vi "MT Set Axis Halt All.vi"() -> (3 "function return":i32)   [LabVIEW 2014, in "MT_API.lvlib"]
doc: "MT_API INT32 __stdcall MT_Set_Axis_Halt_All(void);"
uses:
  MT_API.lvlib
  MT_API.dll
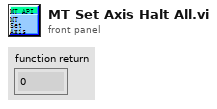
[diagram p1: front panel]
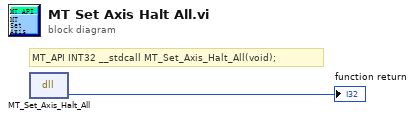
[diagram p0: block diagram]
diagram:
  # "MT_API INT32 __stdcall MT_Set_Axis_Halt_All(void);"
  n1 = dll-call lib="E:/Projects/LabView/MT_API/MT_API.*" fn="MT_Set_Axis_Halt_All"() -> (→"function return":i32)  [unwired: 3 in, 2 out]
